vi "KE622x -- Execute Current Sweep Example.vi"() -> ()   [LabVIEW 2020, in "Keithley 622x.lvlib"]
doc: "Example VI that shows how to set up and execute a linear, log, or list current sweep."
uses:
  Keithley 622x.lvlib
  C/Program Files/National Instruments/LabVIEW 2021/instr.lib/Keithley 622x LV 2009/Typedefs/KE622x -- On Off Control.ctl
  C/Program Files/National Instruments/LabVIEW 2021/instr.lib/Keithley 622x LV 2009/Configure/Source/Typedefs/KE622x -- Source Delay.ctl
  Configure/Source/Typedefs/KE622x -- Current Level.ctl
  C/Program Files/National Instruments/LabVIEW 2021/instr.lib/Keithley 622x LV 2009/Configure/Source/Typedefs/KE622x -- Lin Log Sweep Params.ctl
  C/Program Files/National Instruments/LabVIEW 2021/instr.lib/Keithley 622x LV 2009/Configure/Source/Typedefs/KE622x -- Voltage Limit.ctl
  C/Program Files/National Instruments/LabVIEW 2021/instr.lib/Keithley 622x LV 2009/Configure/Source/Typedefs/KE622x -- List Sweep Step.ctl
  C/Program Files/National Instruments/LabVIEW 2021/instr.lib/Keithley 622x LV 2009/Configure/Source/Typedefs/KE622x -- List Sweep Steps.ctl
  C/Program Files/National Instruments/LabVIEW 2021/instr.lib/Keithley 622x LV 2009/Configure/Source/Typedefs/KE622x -- List Sweep Params.ctl
  C/Program Files/National Instruments/LabVIEW 2021/instr.lib/Keithley 622x LV 2009/Configure/Source/Typedefs/KE622x -- Sweep Type.ctl
  C/Program Files/National Instruments/LabVIEW 2021/instr.lib/Keithley 622x LV 2009/Configure/Trigger/Low Level/Typedefs/KE622x -- Trig Link Line.ctl
  C/Program Files/National Instruments/LabVIEW 2021/instr.lib/Keithley 622x LV 2009/Configure/Trigger/Low Level/Typedefs/KE622x -- Arm Source.ctl
  C/Program Files/National Instruments/LabVIEW 2021/instr.lib/Keithley 622x LV 2009/Configure/Trigger/Low Level/Typedefs/KE622x -- Arm Output Mode.ctl
  C/Program Files/National Instruments/LabVIEW 2021/instr.lib/Keithley 622x LV 2009/Configure/Trigger/Low Level/Typedefs/KE622x -- Arm Timer Interval.ctl
  C/Program Files/National Instruments/LabVIEW 2021/instr.lib/Keithley 622x LV 2009/Configure/Trigger/Typedefs/KE622x -- Arm Layer Params.ctl
  C/Program Files/National Instruments/LabVIEW 2021/instr.lib/Keithley 622x LV 2009/Configure/Trigger/Low Level/Typedefs/KE622x -- Trig Source.ctl
  C/Program Files/National Instruments/LabVIEW 2021/instr.lib/Keithley 622x LV 2009/Configure/Trigger/Low Level/Typedefs/KE622x -- Trig Output Mode.ctl
  C/Program Files/National Instruments/LabVIEW 2021/instr.lib/Keithley 622x LV 2009/Configure/Trigger/Typedefs/KE622x -- Trig Layer Params.ctl
panel:
  in  "Trig Model:  Trig Layer Params":T1
  in  "Trig Model:  Arm Layer Params":T5={"Bypass Arm Layer\nInput Trigger?"=FALSE, "Input Trig Source"=enum."Immediate", "Input Trig Link Line"=enum."1", "Arm Timer Interval (s)"=0.001, "Output Trig Mode"=enum."No Trig Out", "Output Trig Link Line"=enum."1"} {"Arm Timer Interval (s)" min=0.001 max=99999.999 step=0.001 format="%.3f"}
  out "error out":errorcluster
  out "Sweep Completed Normally?":bool
  out "Sweep Timeout?":bool
  out "Sweep Aborted?":bool
  in  "Timeout (msecs)":u32=20000
  in  "Check For SCPI Errors? (T)":bool=TRUE
  in  "KE622x Resource":refnum<visa-resource-name>
  in  "Tab Control":enum32{"Linear or Log Params", "List Params"}(tab)
  in  "Lin Log Sweep Params In":T9={"Sweep Type"=enum."Linear", "Source Delay (s)"=1.0, "Range Method"=enum."Fixed", "Num Sweeps"=enum."Sweep Count", "Sweep Count"=1, "Start Level (A)"=0.0, "Stop Level (A)"=0.1, "Step Level (A)"=0.01, "Num Steps"=11, "Abort On\nCompliance?"=FALSE} {"Num Steps" min=1 max=65535; "Step Level (A)" min=-0.105 max=0.105 format="%.4p"; "Stop Level (A)" min=-0.105 max=0.105 format="%.4p"; "Start Level (A)" min=-0.105 max=0.105 format="%.4p"; "Sweep Count" min=1 max=9999; "Source Delay (s)" min=0.001 max=1000.0 step=0.001 format="%.3f"}
  in  "List Sweep Params":T12={"Abort On\nCompliance?"=TRUE, "List Sweep Steps"=[]} {"List Sweep Steps"."Current Level (A)" min=-0.105 max=0.105 format="%.4p"; "List Sweep Steps"."Source Delay (s)" min=0.001 max=1000.0 step=0.001 format="%.3f"; "List Sweep Steps"."Voltage Limit (V)" min=0.1 max=105.0 step=0.01 format="%.2p"}
  in  "Sweep Type":T16
  # "Input"
  # "Output"
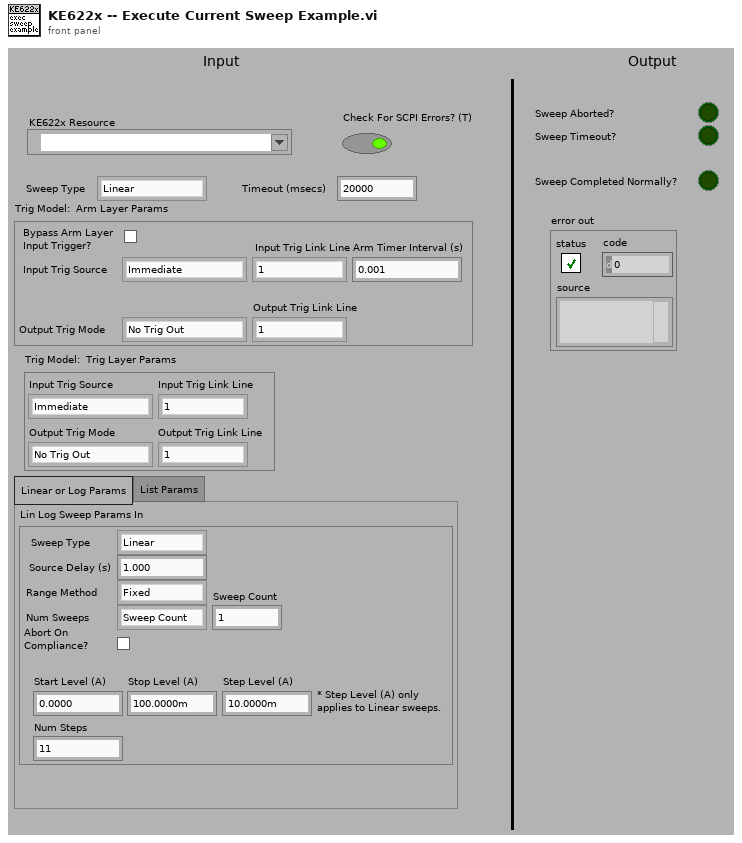
[diagram p1: front panel]
types:
  T1 = typedef "Keithley 622x.lvlib/KE622x -- Trig Layer Params.ctl" = cluster{"Input Trig Source":T2, "Input Trig Link Line":T3, "Output Trig Mode":T4, "Output Trig Link Line":T3}
  T2 = typedef "Keithley 622x.lvlib/KE622x -- Trig Source.ctl" = enum16{"Immediate", "Trigger Link"}
  T3 = typedef "Keithley 622x.lvlib/KE622x -- Trig Link Line.ctl" = enum16{"1", "2", "3", "4", "5", "6"}
  T4 = typedef "Keithley 622x.lvlib/KE622x -- Trig Output Mode.ctl" = enum16{"No Trig Out", "Source Turn On", "After Source Delay"}
  T5 = typedef "Keithley 622x.lvlib/KE622x -- Arm Layer Params.ctl" = cluster{"Bypass Arm Layer\nInput Trigger?":bool, "Input Trig Source":T6, "Input Trig Link Line":T3, "Arm Timer Interval (s)":T7, "Output Trig Mode":T8, "Output Trig Link Line":T3}
  T6 = typedef "Keithley 622x.lvlib/KE622x -- Arm Source.ctl" = enum16{"Immediate", "Bus (*TRG)", "Timer", "Manual", "Trigger Link", "SOT Falling Edge", "SOT Rising Edge", "SOT Either Edge"}
  T7 = typedef "Keithley 622x.lvlib/KE622x -- Arm Timer Interval.ctl" = dbl
  T8 = typedef "Keithley 622x.lvlib/KE622x -- Arm Output Mode.ctl" = enum16{"No Trig Out", "Trig Out On Enter Arm", "Trig Out On Exit Arm"}
  T9 = typedef "Keithley 622x.lvlib/KE622x -- Lin Log Sweep Params.ctl" = cluster{"Sweep Type":enum16{"Linear", "Log", "List"}, "Source Delay (s)":T10, "Range Method":enum16{"Auto", "Best", "Fixed"}, "Num Sweeps":enum16{"Sweep Count", "Infinite"}, "Sweep Count":u32, "Start Level (A)":T11, "Stop Level (A)":T11, "Step Level (A)":T11, "Num Steps":u32, "Abort On\nCompliance?":bool}
  T10 = typedef "Keithley 622x.lvlib/KE622x -- Source Delay.ctl" = dbl
  T11 = typedef "Keithley 622x.lvlib/KE622x -- Current Level.ctl" = dbl
  T12 = typedef "Keithley 622x.lvlib/KE622x -- List Sweep Params.ctl" = cluster{"Abort On\nCompliance?":bool, "List Sweep Steps":T13}
  T13 = typedef "Keithley 622x.lvlib/KE622x -- List Sweep Steps.ctl" = T14[]
  T14 = typedef "Keithley 622x.lvlib/KE622x -- List Sweep Step.ctl" = cluster{"Current Level (A)":T11, "Source Delay (s)":T10, "Voltage Limit (V)":T15}
  T15 = typedef "Keithley 622x.lvlib/KE622x -- Voltage Limit.ctl" = dbl
  T16 = typedef "Keithley 622x.lvlib/KE622x -- Sweep Type.ctl" = enum16{"Linear", "Log", "List"}
  T17 = typedef "Keithley 622x.lvlib/KE622x -- On Off Control.ctl" = enum16{"Off", "On"}
  T18 = typedef "Keithley 622x.lvlib/KE622x -- Op Event Reg State.ctl" = cluster{"B0, CAL:  Instrument Calibrating Event?":bool, "B1, SwpD:  Sweep, Delta, Diff Cond, or Pulse Sweep Complete Event?":bool, "B2, SwpA:  Sweep, Delta, Diff Cond, or Pulse Sweep Aborted Event?":bool, "B3, Swp:  Sweep, Delta, Diff Cond, or Pulse Sweep Sweeping Event?":bool, "B4, WStrt:  KE6221 Wave Mode Started Event?":bool, "B5, Trig:  Waiting For Trigger Event Event?":bool, "B6, Arm:  Waiting For Arm Event Event?":bool, "B7, Wstop:  KE6221 Wave Mode Aborted Event?":bool, "B8, Filt:  Delta Test Started And Filter Settled Event?":bool, "B10, Idle:  Idle State Event?":bool, "B11, RSE:  RS-232 Error Event?":bool}
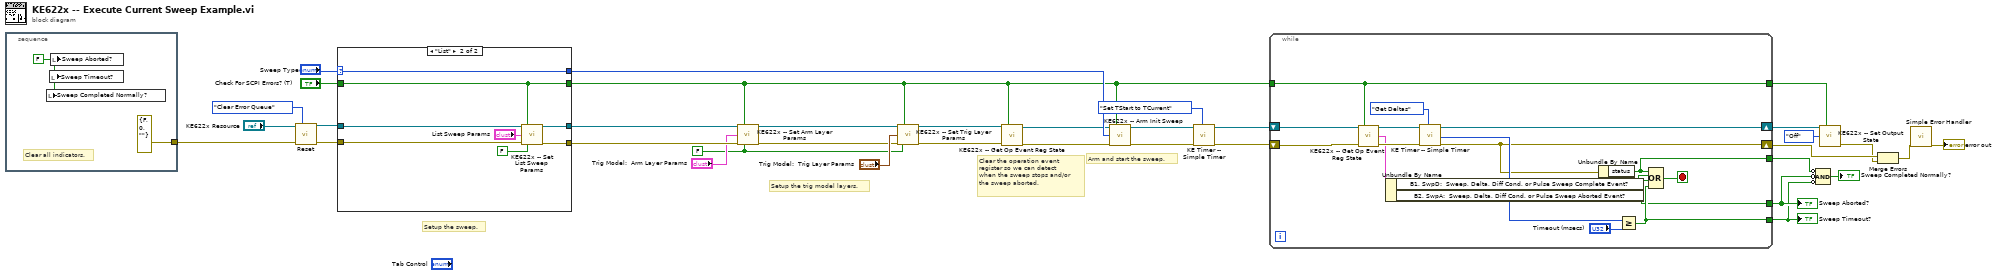
[diagram p0: block diagram]
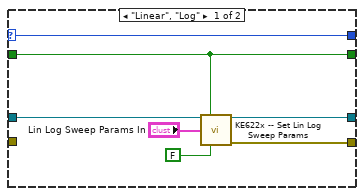
[diagram p2: hidden frame]
diagram:
  w5 = FALSE ("Read Back Set Values? (T)")
  # "Setup the trig model layers."
  # "Clear the operation event\nregister so we can detect\nwhen the sweep stops and/or\nthe sweep aborted."
  # "Arm and start the sweep."
  # "Setup the sweep."
  n1 = stacked-sequence {
    tunnel: [errorcluster {"status"=FALSE, "code"=0, "source"=""} ("error in (no error)")] -> w1
    frame #0 {
      w38 = FALSE ("Sweep Aborted?")
      # "Clear all indicators."
      n2 = local write "Sweep Completed Normally?"(w38) -> ()
      n3 = local write "Sweep Timeout?"(w38) -> ()
      n4 = local write "Sweep Aborted?"(w38) -> ()
    }
  }
  n5 = call "Reset.vi"("VISA resource name"="KE622x Resource", "Error Queue Option"=enum16{"Clear Error Queue", "Error Query"}."Clear Error Queue", "error in (no error)"=w1) -> ("VISA resource name out"=w33:refnum<visa-resource-name>, "error out"=w32:errorcluster)  [unwired: 11 in]
  n6 = case shown="\"List\"" "Sweep Type" {
    selector: "Sweep Type" -> [w40 w46]
    tunnel: w33 -> [w44 w53]
    tunnel: "Check For SCPI Errors? (T)" -> [w39 w47]
    tunnel: [w42 w51] -> w11
    tunnel: [w41 w52] -> w10
    tunnel: w32 -> [_ w49]
    tunnel: [w40 w46] -> w30
    tunnel: [w39 w47] -> w4
    frame "Linear", "Log" {
      n7 = call "KE622x -- Set Lin Log Sweep Params.vi"("Resource In"=w44, "Check For SCPI Errors? (T)"=w39, "Lin Log Sweep Params In"="Lin Log Sweep Params In", "Read Back Set Values? (T)"=FALSE) -> ("Resource Out (dupl)"=w42:refnum<visa-resource-name>, "error out"=w41:errorcluster)  [unwired: 9 in, 1 out]
    }
    frame "List" {
      n8 = call "KE622x -- Set List Sweep Params.vi"("Resource In"=w53, "Check For SCPI Errors? (T)"=w47, "List Sweep Params In"="List Sweep Params", "error in (no error)"=w49, "Read Back Set Values? (T)"=FALSE) -> ("Resource Out (dupl)"=w51:refnum<visa-resource-name>, "error out"=w52:errorcluster)  [unwired: 8 in, 1 out]
    }
  }
  n9 = call "KE622x -- Set Arm Layer Params.vi"("Resource In"=w11, "Check For SCPI Errors? (T)"=w4, "Arm Layer Params In"="Trig Model:  Arm Layer Params", "error in (no error)"=w10, "Read Back Set Values? (T)"=w5) -> ("Resource Out (dupl)"=w7:refnum<visa-resource-name>, "error out"=w6:errorcluster)  [unwired: 8 in, 1 out]
  n10 = call "KE622x -- Set Trig Layer Params.vi"("Resource In"=w7, "Check For SCPI Errors? (T)"=w4, "Trig Layer Params In"="Trig Model:  Trig Layer Params", "error in (no error)"=w6, "Read Back Set Values? (T)"=w5) -> ("Resource Out (dupl)"=w3:refnum<visa-resource-name>, "error out"=w2:errorcluster)  [unwired: 8 in, 1 out]
  n11 = call "KE622x -- Get Op Event Reg State.vi"("VISA Resource In"=w3, "Error Query (T)?"=w4, "error in (no error)"=w2) -> ("VISA Resource Out (dupl)"=w24:refnum<visa-resource-name>, "error out"=w23:errorcluster)  [unwired: 10 in, 1 out]
  n12 = call "KE622x -- Arm Init Sweep.vi"("Resource In"=w24, "Check For SCPI Errors? (T)"=w4, "Sweep Type"=w30, "error in (no error)"=w23) -> ("Resource Out (dupl)"=w29:refnum<visa-resource-name>, "error out"=w28:errorcluster)  [unwired: 10 in]
  n13 = call "KE Timer -- Simple Timer.vi"("Resource In"=w29, "error in (no error)"=w28, "Action"=enum16{"Set TStart to TCurrent", "Get Deltas"}."Set TStart to TCurrent") -> ("Resource Out (dupl)"=w26:refnum<visa-resource-name>, "error out (dupl)"=w25:errorcluster)  [unwired: 7 in, 8 out]
  n14 = while {
    shift-right: [w58] -> w14
    shift-left: w25 -> [w55]
    shift-right: [w59] -> w17
    shift-left: w26 -> [w56]
    tunnel: w4 -> [w54]
    tunnel: [w61] -> w21
    tunnel: [w60] -> w22
    tunnel: [w57] -> w19
    tunnel: [w54] -> w16
    stop <- w62 stop-if-true
    n15 = call "KE622x -- Get Op Event Reg State.vi"("VISA Resource In"=w56, "Error Query (T)?"=w54, "error in (no error)"=w55) -> ("VISA Resource Out (dupl)"=w69:refnum<visa-resource-name>, "KE622x Op Event Reg"=w64:T18, "error out"=w68:errorcluster)  [unwired: 10 in]
    n16 = Unbundle By Name(w64) -> ("B1, SwpD:  Sweep, Delta, Diff Cond, or Pulse Sweep Complete Event?"=w63:bool, "B2, SwpA:  Sweep, Delta, Diff Cond, or Pulse Sweep Aborted Event?"=w60:bool)
    n17 = call "KE Timer -- Simple Timer.vi"("Resource In"=w69, "error in (no error)"=w68, "Action"=enum16{"Set TStart to TCurrent", "Get Deltas"}."Get Deltas") -> ("Resource Out (dupl)"=w59:refnum<visa-resource-name>, "TCurrent - TStart (ms)"=w66:u32, "error out (dupl)"=w58:errorcluster)  [unwired: 7 in, 7 out]
    n18 = Unbundle By Name(w58) -> ("status"=w57:bool)
    n19 = Greater Or Equal?(x=w66, y="Timeout (msecs)") -> (x >= y?=w61:bool)
    n20 = Compound Arithmetic op=OR(w57, w63, w60, w61) -> (w62:bool)
  }
  "Sweep Aborted?" <- w22
  "Sweep Timeout?" <- w21
  n21 = Compound Arithmetic op=AND(invert w19, invert w22, invert w21) -> (→"Sweep Completed Normally?":bool)
  n22 = call "KE622x -- Set Output State.vi"("Resource In"=w17, "Check For SCPI Errors? (T)"=w16, "Output State"=KE622x_--_On_Off_Control."Off") -> ("error out"=w13:errorcluster)  [unwired: 11 in, 1 out]
  n23 = Merge Errors(w14, w13) -> (w12:errorcluster)
  n24 = call <vilib>:"Simple Error Handler.vi"("error in (no error)"=w12) -> ("error out"=→"error out":errorcluster)  [unwired: 4 in, 4 out]
